vi "Set Report Nb_Octet.vi"(8 "error in (no error)":errorcluster caption="entrée d'erreur (pas d'erreur)", 10 "Report Nb_Octet":u16=1 min=1, 11 "Nodon_Send_Command_UART en entrée":refnum<class "Nodon_Send_Command_UART.lvclass">) -> (0 "error out":errorcluster caption="sortie d'erreur", 3 "Nodon_Send_Command_UART en sortie":refnum<class "Nodon_Send_Command_UART.lvclass">)   [LabVIEW 2020, in "Library Test.lvlib" / "Nodon_Send_Command_UART.lvclass"]
uses:
  Nodon_Send_Command_UART.lvclass
  Nodon_Send_Command_UART.lvclass/Nodon_Send_Command_UART.ctl
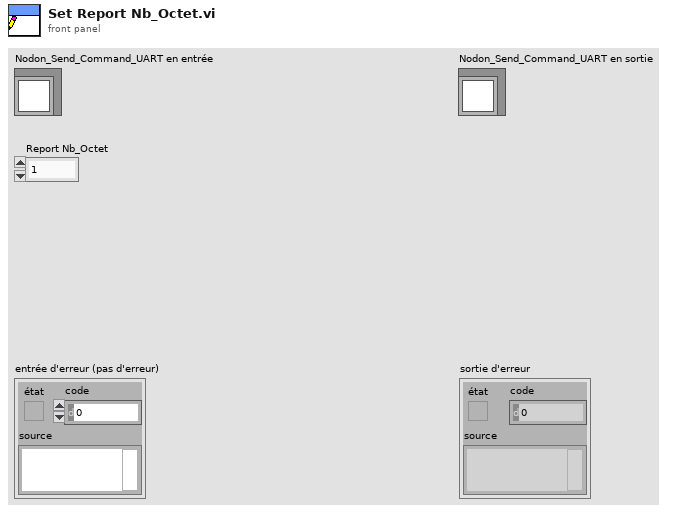
[diagram p1: front panel]
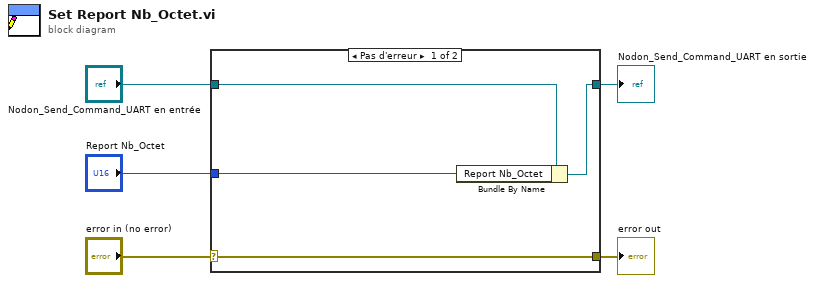
[diagram p0: block diagram]
diagram:
  n1 = case shown="Pas d'erreur" "error in (no error)" {
    selector: "error in (no error)" -> [w9 w10]
    tunnel: [w9 w10] -> w4
    tunnel: [w7 w11] -> w2
    tunnel: "Nodon_Send_Command_UART en entrée" -> [w8 w11]
    tunnel: "Report Nb_Octet" -> [w6 _]
    frame No Error {
      n2 = Bundle By Name(cluster=w8, "Report Nb_Octet"=w6) -> (w7:refnum<class "Nodon_Send_Command_UART.lvclass">)
    }
    frame Error {
    }
  }
  "error out" <- w4
  "Nodon_Send_Command_UART en sortie" <- w2
